vi "Write Dictionary Element.vi"(8 "error in (no error)":errorcluster, 9 "value":variant, 10 "key":string, 11 "Control Experiment":refnum<class "SMO.Control Experiment.lvclass">) -> (0 "error out":errorcluster, 3 "Control Experiment out":refnum<class "SMO.Control Experiment.lvclass">)   [LabVIEW 2019, in "SMO.Control Experiment.lvclass"]
uses:
  SMO.Control Experiment.lvclass
  SMO.Control Experiment.lvclass/SMO.Control Experiment.ctl
  <userlib>/_OpenG.lib/dictionary/dictionary.llb/Dictionary Update (by scalar value)__ogtk.vi
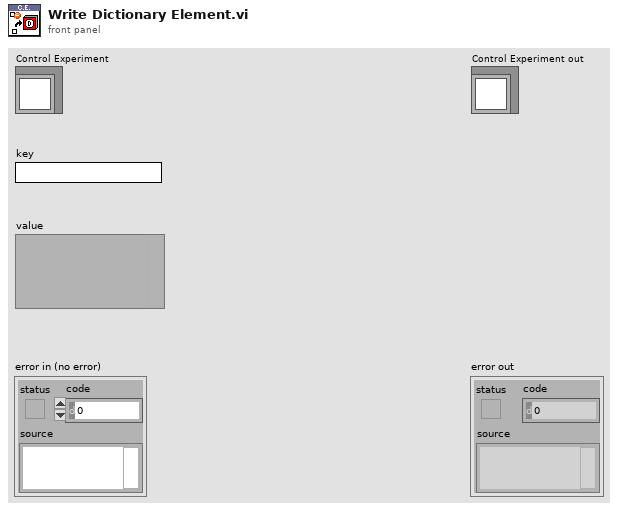
[diagram p1: front panel]
types:
  T1 = typedef "Dictionary Object RefNum__ogtk.ctl" = refnum<k1>
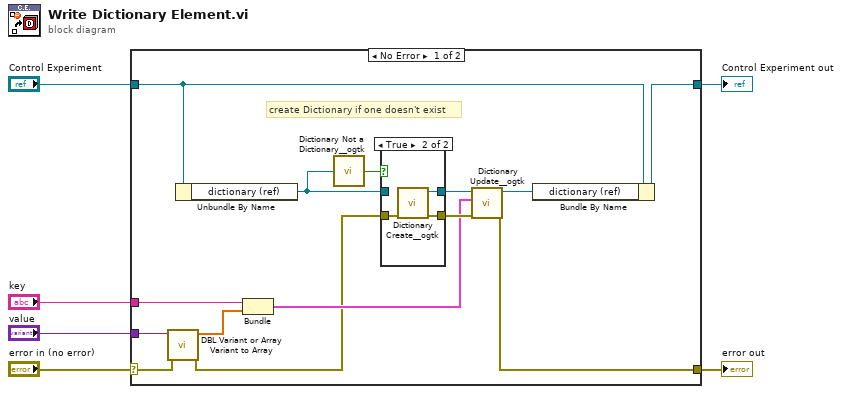
[diagram p0: block diagram]
diagram:
  n1 = case shown="No Error" "error in (no error)" {
    selector: "error in (no error)" -> [w9 w26]
    tunnel: [w16 w26] -> w5
    tunnel: [w20 w27] -> w3
    tunnel: "Control Experiment" -> [w18 w27]
    tunnel: "key" -> [w19 _]
    tunnel: "value" -> [w11 _]
    frame No Error {
      # "create Dictionary if one doesn't exist"
      n2 = call "DBL Variant or Array Variant to Array.vi"("error in (no error)"=w9, "value"=w11) -> ("error out"=w8:errorcluster, "Array"=w10:dbl[])  [unwired: 8 in]
      n3 = Unbundle By Name(w18) -> ("dictionary (ref)"=w7:T1)
      n4 = Bundle("key"=w19, "Array"=w10) -> (w12:cluster{"key":string, "Array":dbl[]})  [unwired: 1 in]
      n5 = call <userlib>:"Dictionary Not a Dictionary__ogtk.vi"("dictionary"=w7) -> ("not a dictionary?"=w14:bool)
      n6 = case shown="True" w14 {
        tunnel: [w22 w25] -> w15
        tunnel: w7 -> [w22 _]
        tunnel: [w21 w24] -> w13
        tunnel: w8 -> [w21 w23]
        frame False {
        }
        frame True {
          n7 = call <userlib>:"Dictionary Create__ogtk.vi"("error in (no error)"=w23) -> ("error out"=w24:errorcluster, "dictionary out"=w25:T1)  [unwired: 9 in]
        }
      }
      n8 = call-poly <userlib>:"Dictionary Update__ogtk.vi"("error in (no error)"=w13, "key-value"=w12, "dictionary"=w15) -> ("error out"=w16:errorcluster, "dictionary out"=w17:T1)  [unwired: 6 in, 1 out]
      n9 = Bundle By Name(cluster=w18, "dictionary (ref)"=w17) -> (w20:refnum<class "SMO.Control Experiment.lvclass">)
    }
    frame Error {
    }
  }
  "error out" <- w5
  "Control Experiment out" <- w3
